vi "Set Reading Buffer.vi"(0 "VISA resource name":refnum<visa-resource-name>="GPIB0::24::INSTR", 3 "Reading Count":i32=10, 11 "error in (no error)":errorcluster) -> (4 "VISA resource name out":refnum<visa-resource-name>="GPIB0::24::INSTR", 15 "error out":errorcluster)   [LabVIEW 2010]
doc: "This Vi allows user to set up the basic source functions. Such as type, level, range, and delay. The VI can be modified to configure other aspects of source."
uses:
  <instrlib>/Keithley 2400/Keithley 24XX.lvlib
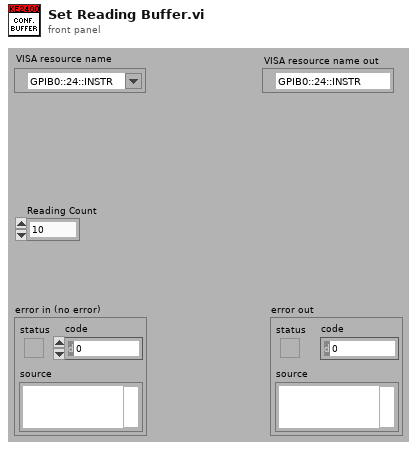
[diagram p1: front panel]
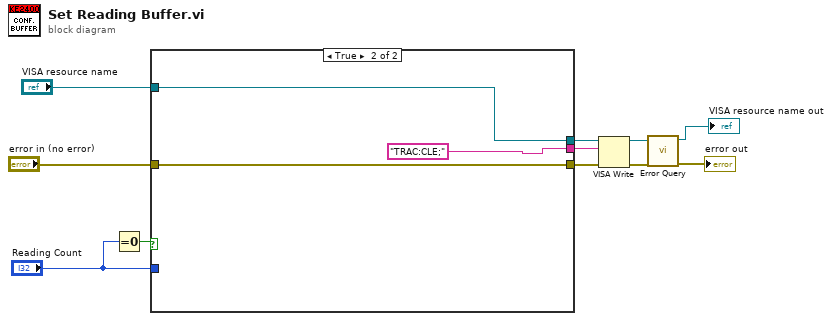
[diagram p0: block diagram]
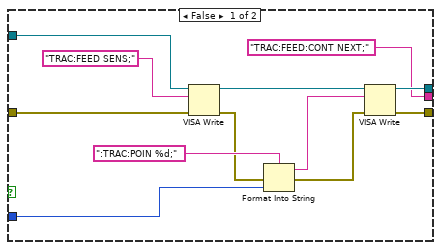
[diagram p2: hidden frame]
diagram:
  n1 = Equal To 0?(x="Reading Count") -> (x = 0?=w1:bool)
  n2 = case shown="True" w1 {
    tunnel: "Reading Count" -> [w20 _]
    tunnel: [w19 w26] -> w9
    tunnel: [w18 w25] -> w8
    tunnel: "VISA resource name" -> [w17 w26]
    tunnel: "error in (no error)" -> [w15 w25]
    tunnel: ["TRAC:FEED:CONT NEXT;" "TRAC:CLE;"] -> w5
    frame False {
      n3 = VISA Write(VISA resource name=w17, write buffer="TRAC:FEED SENS;", error in (no error)=w15) -> (VISA resource name out=w16:refnum<visa-resource-name>, error out=w14:errorcluster)  [unwired: 1 out]
      n4 = Format Into String(format string=":TRAC:POIN %d;", error in=w14, w20) -> (resulting string=w22:string, error out=w21:errorcluster)  [unwired: 1 in]
      n5 = VISA Write(VISA resource name=w16, write buffer=w22, error in (no error)=w21) -> (VISA resource name out=w19:refnum<visa-resource-name>, error out=w18:errorcluster)  [unwired: 1 out]
    }
    frame True {
    }
  }
  n6 = VISA Write(VISA resource name=w9, write buffer=w5, error in (no error)=w8) -> (VISA resource name out=w4:refnum<visa-resource-name>, error out=w3:errorcluster)  [unwired: 1 out]
  n7 = call <instrlib>:"Error Query.vi"("error in (no error)"=w3, "VISA resource name"=w4) -> ("error out"=→"error out":errorcluster, "VISA resource name out"=→"VISA resource name out":refnum<visa-resource-name>)  [unwired: 6 in, 2 out]
